vi "disk_closeDiskTemplate.vi"(8 "error in (no error)":errorcluster, 11 "DiskTemplate in":T1={"XMLRef"=[refnum, refnum, refnum, refnum, refnum, refnum], "ZipPath"=path "", "MetaFile"={"Ref"=refnum, "NextRow"=0, "NextPosition"=0, "Block"=[]}, "TempFolder"=path ""}) -> (0 "error out":errorcluster)   [LabVIEW 2020, in "NI_ExcelFile.lvlib"]
uses:
  <vilib>/express/express shared/NI_ExcelFile/NI_ExcelFile.lvlib
  <vilib>/express/express shared/NI_ExcelFile/Ctrls/disk_TemplateFile.ctl
  <vilib>/express/express shared/NI_ExcelFile/Ctrls/meta_file.ctl
  <vilib>/express/express shared/NI_ExcelFile/Ctrls/meta_Block.ctl
  <vilib>/express/express shared/NI_ExcelFile/Ctrls/meta_BlockType.ctl
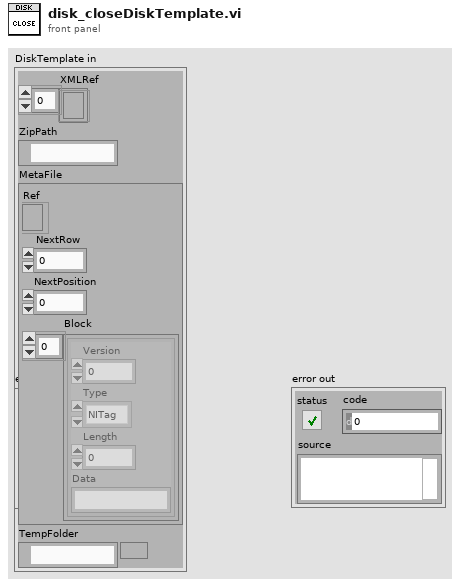
[diagram p1: front panel]
types:
  T1 = typedef "NI_ExcelFile.lvlib/disk_TemplateFile.ctl" = cluster{"XMLRef":refnum<file>[], "ZipPath":path, "MetaFile":T2, "TempFolder":path}
  T2 = typedef "NI_ExcelFile.lvlib/meta_file.ctl" = cluster{"Ref":refnum<file>, "NextRow":i32, "NextPosition":i64, "Block":T3[]}
  T3 = typedef "NI_ExcelFile.lvlib/meta_Block.ctl" = cluster{"Version":u16, "Type":T4, "Length":i32, "Data":string}
  T4 = typedef "NI_ExcelFile.lvlib/meta_BlockType.ctl" = enum16{"NITag", "File", "Column"}
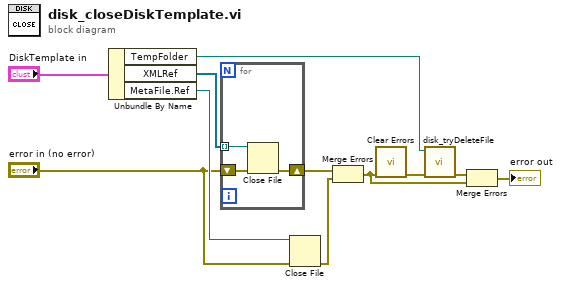
[diagram p0: block diagram]
diagram:
  n1 = Unbundle By Name("DiskTemplate in") -> ("TempFolder"=w5:path, "XMLRef"=w10:refnum<file>[], "MetaFile.Ref"=w9:refnum<file>)
  n2 = for {
    tunnel: w10 -> [w12] mode=indexing
    shift-right: [w14] -> w8
    shift-left: "error in (no error)" -> [w13]
    n3 = Close File(refnum=w12, error in=w13) -> (error out=w14:errorcluster)  [unwired: 1 out]
  }
  n4 = Close File(refnum=w9, error in="error in (no error)") -> (error out=w7:errorcluster)  [unwired: 1 out]
  n5 = Merge Errors(w8, w7) -> (w3:errorcluster)
  n6 = call <vilib>:"Clear Errors.vi"("error in (no error)"=w3) -> ("error out"=w4:errorcluster)  [unwired: 5 in, 1 out]
  n7 = call <vilib>:"disk_tryDeleteFile.vi"("error in (no error)"=w4, "path"=w5) -> ("error out"=w2:errorcluster)  [unwired: 9 in]
  n8 = Merge Errors(w2, w3) -> (→"error out":errorcluster)
